vi "CAL_Power_L.vi"(0 "stride?":bool, 2 "Positive Power":sgl[](array[numeric]), 3 "출력 클러스터 2":T1, 4 "Period_L":sgl) -> (10 "출력 클러스터 3":T1)   [LabVIEW 2019]
panel:
  in  "Negative Powe":sgl[](array[numeric])
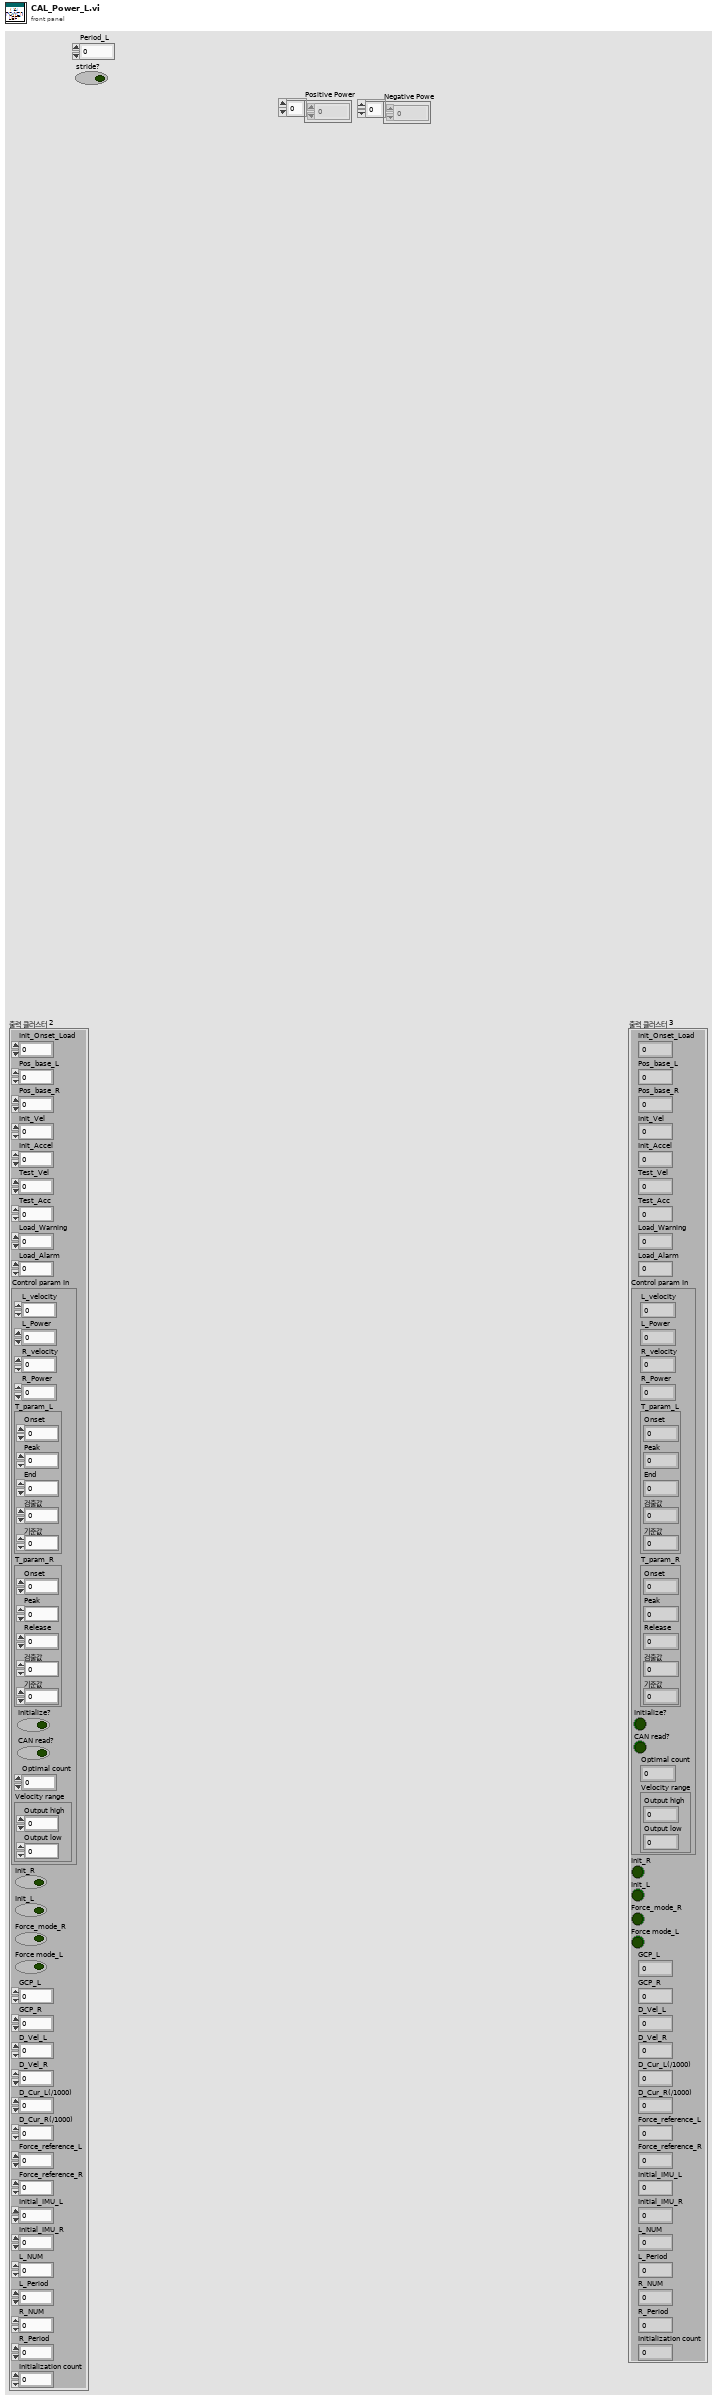
[diagram p1: front panel]
types:
  T1 = cluster{"Init_Onset_Load":sgl, "Pos_base_L":sgl, "Pos_base_R":sgl, "Init_Vel":i32, "Init_Accel":u32, "Test_Vel":i32, "Test_Acc":u32, "Load_Warning":sgl, "Load_Alarm":sgl, "Control param In":cluster{"L_velocity":u32, "L_Power":sgl, "R_velocity":u32, "R_Power":sgl, "T_param_L":cluster{"Onset":sgl, "Peak":sgl, "End":sgl, "검출값":sgl, "기준값":sgl}, "T_param_R":cluster{"Onset":sgl, "Peak":sgl, "Release":sgl, "검출값":sgl, "기준값":sgl}, "Initialize?":bool, "CAN read?":bool, "Optimal count":i32, "Velocity range":cluster{"Output high":dbl, "Output low":dbl}}, "Init_R":bool, "Init_L":bool, "Force_mode_R":bool, "Force mode_L":bool, "GCP_L":sgl, "GCP_R":sgl, "D_Vel_L":sgl, "D_Vel_R":sgl, "D_Cur_L(/1000)":sgl, "D_Cur_R(/1000)":sgl, "Force_reference_L":sgl, "Force_reference_R":sgl, "Initial_IMU_L":sgl, "Initial_IMU_R":sgl, "L_NUM":u32, "L_Period":i16, "R_NUM":u32, "R_Period":i16, "Initialization count":i32}
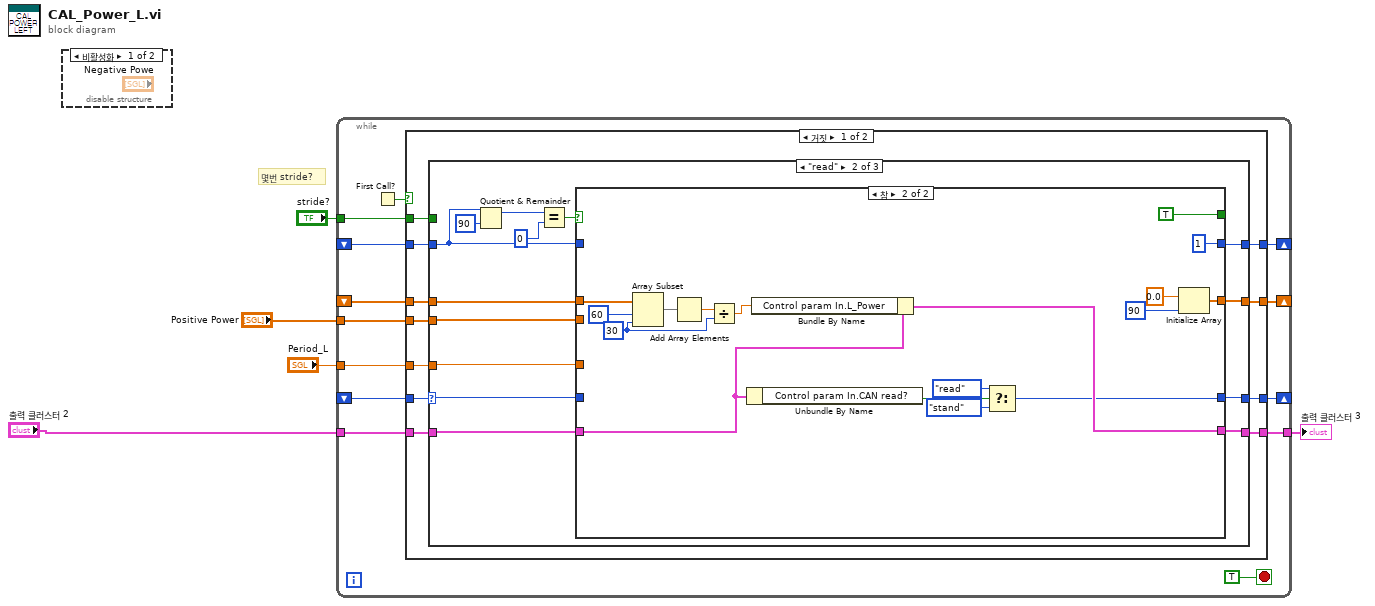
[diagram p0: block diagram]
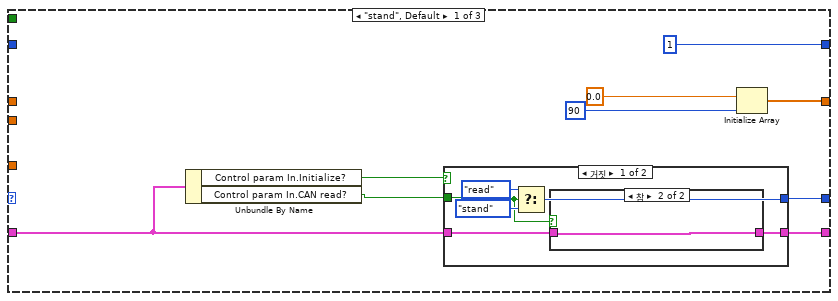
[diagram p2: hidden frame]
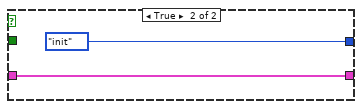
[diagram p4: hidden frame]
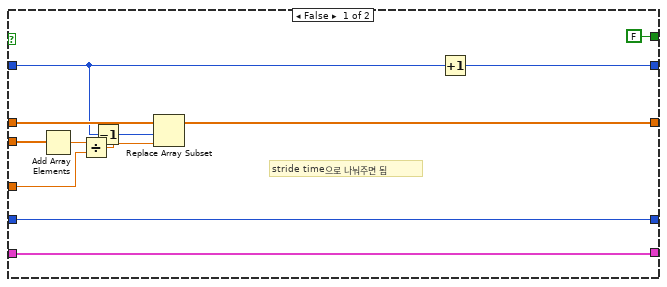
[diagram p5: hidden frame]
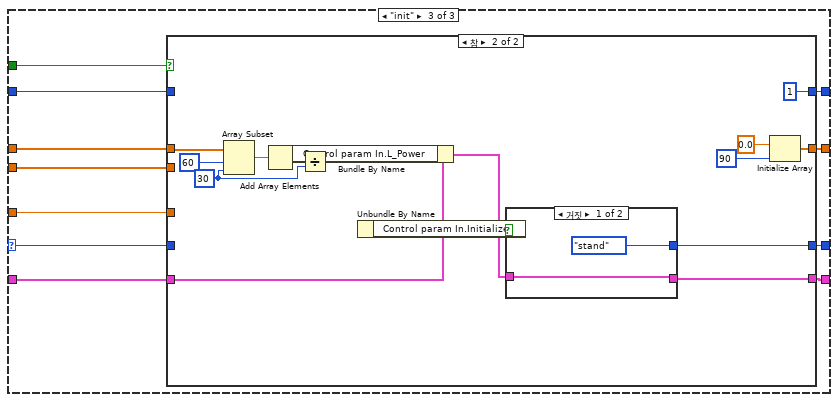
[diagram p6: hidden frame]
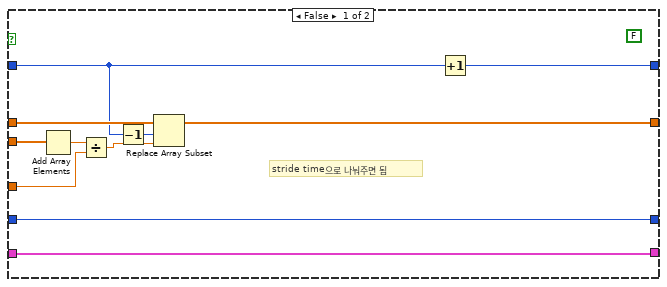
[diagram p7: hidden frame]
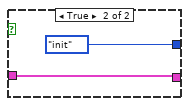
[diagram p8: hidden frame]
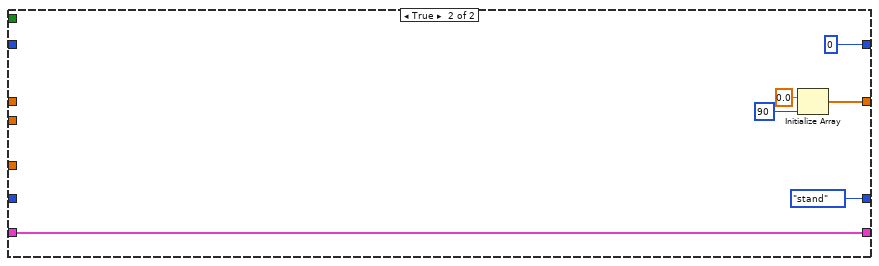
[diagram p9: hidden frame]
diagram:
  # "몇번 stride?"
  n1 = disable-structure shown="비활성화" {
    frame Disabled {
    }
    frame Enabled {
    }
  }
  n2 = while {
    tunnel: "Positive Power" -> [w12]
    shift-right: [w16] -> _
    shift-left: _ -> [w15]
    shift-right: [w14] -> _
    shift-left: _ -> [w13]
    tunnel: "출력 클러스터 2" -> [w11]
    tunnel: [w10] -> w1
    tunnel: "stride?" -> [w9]
    tunnel: "Period_L" -> [w8]
    shift-right: [w7] -> _
    shift-left: _ -> [w6]
    stop <- TRUE stop-if-true
    n3 = First Call?() -> (First Call?: T/F=w17:bool)
    n4 = case shown="거짓" w17 {
      tunnel: [w29 0] -> w16
      tunnel: w15 -> [w28 _]
      tunnel: [w25 w135] -> w14
      tunnel: w13 -> [w27 _]
      tunnel: w12 -> [w26 _]
      tunnel: w11 -> [w21 w134]
      tunnel: [w24 w134] -> w10
      tunnel: w9 -> [w23 _]
      tunnel: w8 -> [w22 _]
      tunnel: [w20 enum16{"stand", "init", "read"}."stand" ("CAN")] -> w7
      tunnel: w6 -> [w19 _]
      frame False {
        n5 = case shown="\"read\"" w19 {
          selector: w19 -> [_ w59 w93]
          tunnel: [1 w57 w102] -> w29
          tunnel: w28 -> [_ w50 w101]
          tunnel: w27 -> [_ w62 w100]
          tunnel: w26 -> [_ w61 w99]
          tunnel: [w35 w58 w98] -> w25
          tunnel: [w30 w55 w97] -> w24
          tunnel: w23 -> [_ _ w96]
          tunnel: w22 -> [_ w60 w95]
          tunnel: w21 -> [w31 w49 w94]
          tunnel: [w34 w56 w92] -> w20
          frame "stand", Default {
            n6 = Unbundle By Name(w31) -> ("Control param In.Initialize?"=w33:bool, "Control param In.CAN read?"=w32:bool)
            n7 = case shown="거짓" w33 {
              tunnel: [w42 enum16{"stand", "init", "read"}."init" ("CAN")] -> w34
              tunnel: w32 -> [w41 _]
              tunnel: w31 -> [w40 w47]
              tunnel: [w39 w47] -> w30
              frame False {
                n8 = Select(t=enum16{"stand", "init", "read"}."read" ("CAN"), s=w41, f=enum16{"stand", "init", "read"}."stand" ("CAN")) -> (s? t:f=w42:enum16{"stand", "init", "read"})
                n9 = case shown="참" w41 {
                  tunnel: w40 -> [w45 w46]
                  tunnel: [w45 w46] -> w39
                  frame False {
                  }
                  frame True {
                  }
                }
              }
              frame True {
              }
            }
            n10 = Initialize Array(sgl 0.0 ("원소"), 90 ("차원 크기")) -> (w35:sgl[])
          }
          frame "read" {
            n11 = Quotient & Remainder(x=w50, y=u32 90) -> (x-y*floor(x/y)=w53:u32)  [unwired: 1 out]
            n12 = Equal?(x=w53, y=u32 0) -> (x = y?=w51:bool)
            n13 = case shown="참" w51 {
              tunnel: [w74 1 ("y")] -> w57
              tunnel: w50 -> [w64 _]
              tunnel: w62 -> [w73 w85]
              tunnel: w61 -> [w69 _]
              tunnel: [w72 w88] -> w58
              tunnel: [w71 w87] -> w55
              tunnel: w49 -> [w71 w77]
              tunnel: [FALSE TRUE] -> _
              tunnel: w60 -> [w67 _]
              tunnel: w59 -> [w65 _]
              tunnel: [w65 w80] -> w56
              frame False {
                # "stride time으로 나눠주면 됨"
                n14 = Add Array Elements(numeric array=w69) -> (sum=w68:sgl)
                n15 = Divide(x=w68, y=w67) -> (x/y=w66:sgl)
                n16 = Decrement(x=w64) -> (x-1=w63:i32)
                n17 = Replace Array Subset(array=w73, new element=w66, index=w63) -> (w72:sgl[])
                n18 = Increment(x=w64) -> (x+1=w74:i32)
              }
              frame True {
                w81 = 30 ("길이")
                n19 = Array Subset(array=w85, index=60 ("인덱스"), length=w81) -> (w83:sgl[])
                n20 = Add Array Elements(numeric array=w83) -> (sum=w82:sgl)
                n21 = Divide(x=w82, y=w81) -> (x/y=w75:sgl)
                n22 = Unbundle By Name(w77) -> ("Control param In.CAN read?"=w76:bool)
                n23 = Bundle By Name(cluster=w77, "Control param In.L_Power"=w75) -> (w87:T1)
                n24 = Select(t=enum16{"stand", "init", "read"}."read" ("CAN"), s=w76, f=enum16{"stand", "init", "read"}."stand" ("CAN")) -> (s? t:f=w80:enum16{"stand", "init", "read"})
                n25 = Initialize Array(sgl 0.0 ("원소"), 90 ("차원 크기")) -> (w88:sgl[])
              }
            }
          }
          frame "init" {
            n26 = case shown="참" w96 {
              tunnel: [w113 1 ("y")] -> w102
              tunnel: w101 -> [w104 _]
              tunnel: w100 -> [w112 w124]
              tunnel: w99 -> [w109 _]
              tunnel: [w111 w125] -> w98
              tunnel: [w110 w115] -> w97
              tunnel: w94 -> [w110 w118]
              tunnel: w95 -> [w107 _]
              tunnel: w93 -> [w105 _]
              tunnel: [w105 w119] -> w92
              frame False {
                (unwired) FALSE
                # "stride time으로 나눠주면 됨"
                n27 = Add Array Elements(numeric array=w109) -> (sum=w108:sgl)
                n28 = Divide(x=w108, y=w107) -> (x/y=w106:sgl)
                n29 = Decrement(x=w104) -> (x-1=w103:i32)
                n30 = Replace Array Subset(array=w112, new element=w106, index=w103) -> (w111:sgl[])
                n31 = Increment(x=w104) -> (x+1=w113:i32)
              }
              frame True {
                w120 = 30 ("길이")
                n32 = Array Subset(array=w124, index=60 ("인덱스"), length=w120) -> (w122:sgl[])
                n33 = Add Array Elements(numeric array=w122) -> (sum=w121:sgl)
                n34 = Divide(x=w121, y=w120) -> (x/y=w114:sgl)
                n35 = Bundle By Name(cluster=w118, "Control param In.L_Power"=w114) -> (w116:T1)
                n36 = Unbundle By Name(w118) -> ("Control param In.Initialize?"=w117:bool)
                n37 = case shown="거짓" w117 {
                  tunnel: [enum16{"stand", "init", "read"}."stand" ("CAN") enum16{"stand", "init", "read"}."init" ("CAN")] -> w119
                  tunnel: w116 -> [w129 w131]
                  tunnel: [w129 w131] -> w115
                  frame False {
                  }
                  frame True {
                  }
                }
                n38 = Initialize Array(sgl 0.0 ("원소"), 90 ("차원 크기")) -> (w125:sgl[])
              }
            }
          }
        }
      }
      frame True {
        n39 = Initialize Array(sgl 0.0 ("원소"), 90 ("차원 크기")) -> (w135:sgl[])
      }
    }
  }
  "출력 클러스터 3" <- w1
